vi "Get Next.vi"(0 "Conditional in":refnum<class "Conditional.lvclass">, 1 "Linked List Ref":refnum<data-value>, 5 "Active Unique ID":string, 9 "Active Element Index":i32, 11 "error in (no error)":errorcluster) -> (3 "Linked List Ref out":refnum<data-value>, 4 "Executioner out":refnum<class "Executioner.lvclass">, 6 "Active Unique ID out":string, 8 "Test Executive Ref out":refnum<data-value>, 10 "Active Element Index out":i32, 12 "Found":bool, 13 "Complete":bool, 14 "Stop":bool, 15 "error out":errorcluster)   [LabVIEW 2017, in "Custom Type Test Executive.lvlib" / "Conditional.lvclass"]
uses:
  <vilib>/gpm_packages/@cs/test-executive/Source/Custom Type Test Executive/Conditional/Conditional.lvclass
  C:/Program Files/National Instruments/LabVIEW 2017/vi.lib/gpm_packages/@cs/test-executive/Source/Test Executive/Executioner/Executioner.lvclass
  <vilib>/gpm_packages/@cs/test-executive/Source/Test Executive/Executioner/Executioner.lvclass
  <vilib>/gpm_packages/@cs/linked-list/Source/Linked List/ILinkedList/ILinked List.lvclass
  <vilib>/gpm_packages/@cs/test-executive/Source/Test Executive/ITestExecutive/ITest Executive.lvclass
  <vilib>/gpm_packages/@cs/data-type-serializer/source/String/String.lvclass/String.ctl
  <vilib>/gpm_packages/@cs/data-type-serializer/source/Boolean/Boolean.lvclass/Boolean.ctl
  <vilib>/gpm_packages/@cs/run-time-assertions/Source/Assert/Assert.lvclass
  <vilib>/gpm_packages/@cs/data-type-serializer/source/Assertion/Assertion.lvclass/Assertion.ctl
  3077af34-4ef3-437c-b8d8-6eac68132344.vi
  9cbd8125-b855-42de-ba09-e02fd7405d46.vi
  3190a705-8440-4941-9536-4da4aa80a172.vi
  cabaf482-ba4b-46e4-9c21-873f7cc35bd3.vi
  ea6f5d10-5cf1-43e9-b612-598c02a8f936.vi
  9307d838-b7ae-42de-b3ed-71b38e2b7019.vi
  380485d8-fc70-4f46-821f-d05b1d9706b5.vi
  58626fd2-b79f-420a-b1ac-c7491086ee9c.vi
  da5c0a25-912c-45e8-99a2-8536258bb53a.vi
  193c418e-592a-406e-a7dd-eacb90f55738.vi
  <vilib>/gpm_packages/@cs/data-type-serializer/source/Boolean/Boolean.lvclass
  C:/Program Files/National Instruments/LabVIEW 2017/vi.lib/gpm_packages/@cs/data-type-serializer/source/Data Type/Data Type.lvclass
  <vilib>/gpm_packages/@cs/data-type-serializer/source/Assertion/Assertion.lvclass
  <vilib>/gpm_packages/@cs/data-type-serializer/source/String/String.lvclass
  <vilib>/gpm_packages/@cs/linked-list/Source/Linked List/Linked List Ref/Linked List Ref.lvclass
  <vilib>/gpm_packages/@cs/test-executive/Source/Test Executive/Conditional/Conditional.lvclass
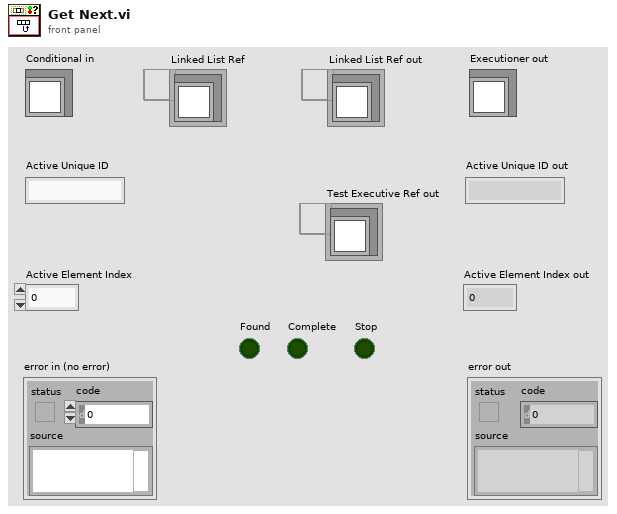
[diagram p1: front panel]
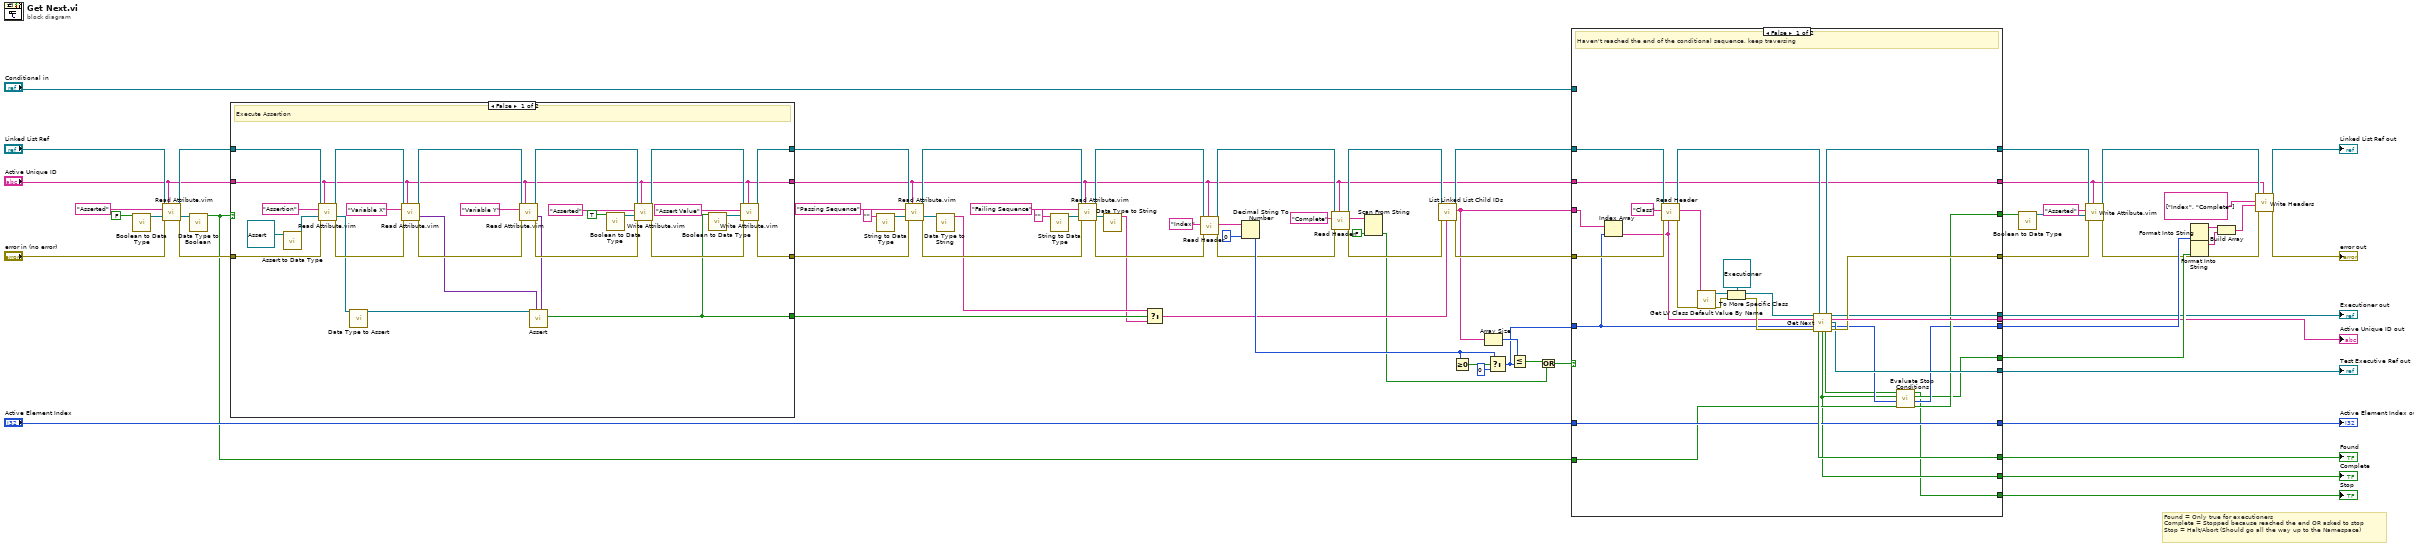
[diagram p0: block diagram]
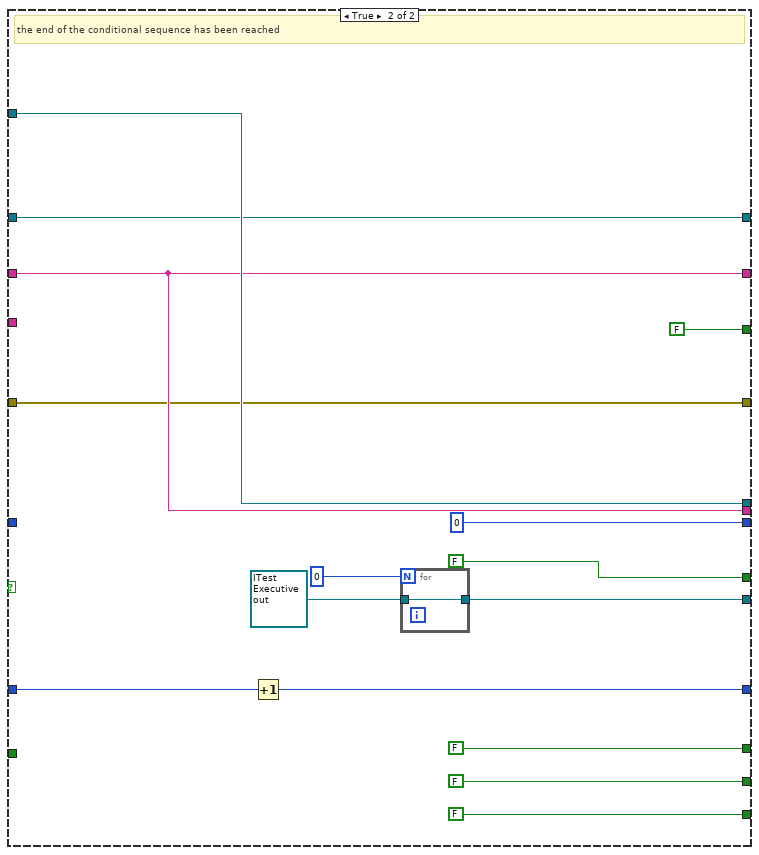
[diagram p2: hidden frame]
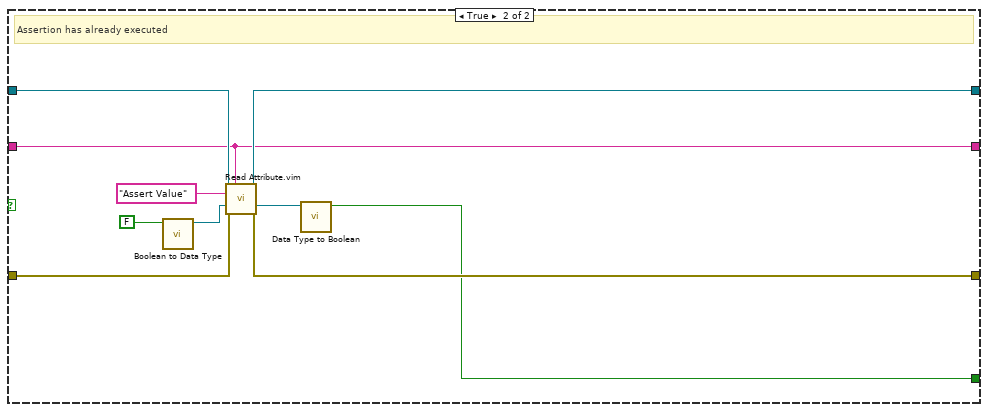
[diagram p3: hidden frame]
diagram:
  # "Found = Only true for executioners\nComplete = Stopped because reached the end OR asked to stop\nStop = Halt/Abort (Should go all the way up to the Namespace)"
  n1 = call <vilib>:"Boolean to Data Type.vi"("Boolean"=FALSE) -> ("Boolean out"=w13:refnum<class "Boolean.lvclass">)  [unwired: 9 in, 1 out]
  n2 = call "Read Attribute.vim"("Linked List Ref"="Linked List Ref", "Linked List ID"="Active Unique ID", "Attribute Name"="Asserted", "Type"=w13, "error in (no error)"="error in (no error)") -> ("Linked List Ref out"=w74:refnum<data-value>, "Attribute"=w12:refnum<class "Boolean.lvclass">, "error out"=w73:errorcluster)  [unwired: 5 in, 3 out]
  n3 = call <vilib>:"Data Type to Boolean.vi"("Data Type"=w12) -> ("Boolean out"=w11:bool)  [unwired: 9 in, 1 out]
  n4 = case shown="False" w11 {
    tunnel: "Active Unique ID" -> [w86 w108]
    tunnel: [w94 w111] -> w71
    tunnel: [w92 w109] -> w72
    tunnel: w74 -> [w98 w112]
    tunnel: w73 -> [w97 w110]
    tunnel: [w77 w106] -> w66
    tunnel: [w86 w108] -> w39
    frame False {
      # "Execute Assertion"
      n5 = call <vilib>:"Assert to Data Type.vi"("Assert"=refnum<class "Assert.lvclass"> refnum ("Run Time Assertions.lvlib:Assert.lvclass")) -> ("Assert out"=w82:refnum<class "Assertion.lvclass">)  [unwired: 9 in, 1 out]
      n6 = call "Read Attribute.vim"("Linked List Ref"=w98, "Linked List ID"=w86, "Attribute Name"="Assertion", "Type"=w82, "error in (no error)"=w97) -> ("Linked List Ref out"=w102:refnum<data-value>, "Attribute"=w81:refnum<class "Assertion.lvclass">, "error out"=w101:errorcluster)  [unwired: 5 in, 3 out]
      n7 = call <vilib>:"Data Type to Assert.vi"("Data Type"=w81) -> ("Assert"=w80:refnum<class "Assert.lvclass">)  [unwired: 9 in, 1 out]
      n8 = call "Read Attribute.vim"("Linked List Ref"=w102, "Linked List ID"=w86, "Attribute Name"="Variable X", "error in (no error)"=w101) -> ("Linked List Ref out"=w89:refnum<data-value>, "Attribute"=w85:variant, "error out"=w90:errorcluster)  [unwired: 6 in, 3 out]
      n9 = call "Read Attribute.vim"("Linked List Ref"=w89, "Linked List ID"=w86, "Attribute Name"="Variable Y", "error in (no error)"=w90) -> ("Linked List Ref out"=w87:refnum<data-value>, "Attribute"=w84:variant, "error out"=w88:errorcluster)  [unwired: 6 in, 3 out]
      n10 = call-dynamic "Assert.vi"("Variable Y"=w84, "Variable X"=w85, "Assert in"=w80) -> ("Assert?"=w77:bool)  [unwired: 8 in]
      n11 = call <vilib>:"Boolean to Data Type.vi"("Boolean"=TRUE) -> ("Boolean out"=w78:refnum<class "Boolean.lvclass">)  [unwired: 9 in, 1 out]
      n12 = call "Write Attribute.vim"("Linked List ID"=w86, "error in (no error)"=w88, "Attribute"=w78, "Attribute Name"="Asserted", "Linked List Ref"=w87) -> ("error out"=w93:errorcluster, "Linked List Ref out"=w95:refnum<data-value>)  [unwired: 3 in, 2 out]
      n13 = call <vilib>:"Boolean to Data Type.vi"("Boolean"=w77) -> ("Boolean out"=w76:refnum<class "Boolean.lvclass">)  [unwired: 9 in, 1 out]
      n14 = call "Write Attribute.vim"("Linked List ID"=w86, "error in (no error)"=w93, "Attribute"=w76, "Attribute Name"="Assert Value", "Linked List Ref"=w95) -> ("error out"=w92:errorcluster, "Linked List Ref out"=w94:refnum<data-value>)  [unwired: 3 in, 2 out]
    }
    frame True {
      # "Assertion has already executed"
      n15 = call <vilib>:"Boolean to Data Type.vi"("Boolean"=FALSE) -> ("Boolean out"=w104:refnum<class "Boolean.lvclass">)  [unwired: 9 in, 1 out]
      n16 = call "Read Attribute.vim"("Linked List Ref"=w112, "Linked List ID"=w108, "Attribute Name"="Assert Value", "Type"=w104, "error in (no error)"=w110) -> ("Linked List Ref out"=w111:refnum<data-value>, "Attribute"=w107:refnum<class "Boolean.lvclass">, "error out"=w109:errorcluster)  [unwired: 5 in, 3 out]
      n17 = call <vilib>:"Data Type to Boolean.vi"("Data Type"=w107) -> ("Boolean out"=w106:bool)  [unwired: 9 in, 1 out]
    }
  }
  n18 = call <vilib>:"String to Data Type.vi"("String"="") -> ("Boolean out"=w9:refnum<class "String.lvclass">)  [unwired: 9 in, 1 out]
  n19 = call "Read Attribute.vim"("Linked List Ref"=w71, "Linked List ID"=w39, "Attribute Name"="Passing Sequence", "Type"=w9, "error in (no error)"=w72) -> ("Linked List Ref out"=w68:refnum<data-value>, "Attribute"=w8:refnum<class "String.lvclass">, "error out"=w67:errorcluster)  [unwired: 5 in, 3 out]
  n20 = call <vilib>:"Data Type to String.vi"("Data Type"=w8) -> ("String out"=w7:string)  [unwired: 9 in, 1 out]
  n21 = call <vilib>:"String to Data Type.vi"("String"="") -> ("Boolean out"=w5:refnum<class "String.lvclass">)  [unwired: 9 in, 1 out]
  n22 = call "Read Attribute.vim"("Linked List Ref"=w68, "Linked List ID"=w39, "Attribute Name"="Failing Sequence", "Type"=w5, "error in (no error)"=w67) -> ("Linked List Ref out"=w65:refnum<data-value>, "Attribute"=w4:refnum<class "String.lvclass">, "error out"=w64:errorcluster)  [unwired: 5 in, 3 out]
  n23 = call <vilib>:"Data Type to String.vi"("Data Type"=w4) -> ("String out"=w3:string)  [unwired: 9 in, 1 out]
  n24 = Select(t=w7, s=w66, f=w3) -> (s? t:f=w54:string)
  n25 = call <vilib>:"Read Header.vi"("Linked List ID"=w39, "error in (no error)"=w64, "Header Name"="Index" ("Attribute Name"), "Linked List Ref"=w65) -> ("error out"=w38:errorcluster, "Header Value"=w51:string, "Linked List Ref out"=w41:refnum<data-value>)  [unwired: 4 in, 1 out]
  n26 = Decimal String To Number(string=w51, default (0L)=0 ("Attribute")) -> (number=w60:i32)  [unwired: 1 in, 1 out]
  n27 = call <vilib>:"Read Header.vi"("Linked List ID"=w39, "error in (no error)"=w38, "Header Name"="Complete" ("Attribute Name"), "Linked List Ref"=w41) -> ("error out"=w37:errorcluster, "Header Value"=w43:string, "Linked List Ref out"=w40:refnum<data-value>)  [unwired: 4 in, 1 out]
  n28 = Scan From String(input string=w43, default 1=FALSE) -> (output 1=w35:bool)  [unwired: 3 in, 3 out]
  n29 = call <vilib>:"List Linked List Child IDs.vi"("Linked List ID"=w54, "error in (no error)"=w37, "Linked List Ref"=w40) -> ("error out"=w58:errorcluster, "Child IDs"=w57:string[], "Linked List Ref out"=w59:refnum<data-value>)  [unwired: 6 in]
  n30 = Greater Or Equal To 0?(x=w60) -> (x >= 0?=w63:bool)
  n31 = Array Size(array=w57) -> (size(s)=w61:i32)
  n32 = Select(t=w60, s=w63, f=0) -> (s? t:f=w56:i32)
  n33 = Less Or Equal?(x=w61, y=w56) -> (x <= y?=w45:bool)
  n34 = Or(x=w45, y=w35) -> (x .or. y?=w36:bool)
  n35 = case shown="False" w36 {
    tunnel: [w134 w146] -> w32
    tunnel: w59 -> [w136 w146]
    tunnel: [w130 w145] -> w30
    tunnel: w58 -> [w138 w145]
    tunnel: w57 -> [w127 _]
    tunnel: w56 -> [w126 _]
    tunnel: [w118 0 ("Active Element Index out")] -> w55
    tunnel: [w122 w155] -> w16
    tunnel: [w133 w151] -> w15
    tunnel: [w132 FALSE ("Found")] -> w20
    tunnel: [w117 FALSE] -> w21
    tunnel: [w114 FALSE] -> w22
    tunnel: "Conditional in" -> [_ w155]
    tunnel: w39 -> [w129 w151]
    tunnel: [w129 w151] -> w29
    tunnel: "Active Element Index" -> [w128 w153]
    tunnel: [w128 w152] -> w19
    tunnel: [w116 FALSE ("Complete")] -> w53
    tunnel: [w124 w147] -> w18
    tunnel: [w120 FALSE] -> w1
    tunnel: w11 -> [w121 _]
    frame False {
      # "Haven't reached the end of the conditional sequence, keep traversing"
      n36 = Index Array(array=w127, index=w126) -> (element=w125:string)
      n37 = call <vilib>:"Read Header.vi"("Linked List ID"=w125, "error in (no error)"=w138, "Header Name"="Class", "Linked List Ref"=w136) -> ("error out"=w131:errorcluster, "Header Value"=w143:string, "Linked List Ref out"=w135:refnum<data-value>)  [unwired: 4 in, 1 out]
      n38 = call <vilib>:"Get LV Class Default Value By Name.vi"("error in (no error)"=w131, "class name"=w143) -> ("error out"=w139:errorcluster, "object"=w142:refnum<class>)  [unwired: 8 in]
      n39 = To More Specific Class(target class=refnum<class "Executioner.lvclass"> refnum ("Test Executive.lvlib:Executioner.lvclass"), reference=w142, error in=w139) -> (specific class reference=w123:refnum<class "Executioner.lvclass">, error out=w140:errorcluster)
      n40 = call-dynamic "Get Next.vi"("Executioner in"=w123, "Linked List Ref"=w135, "Active Unique ID"=w125, "Active Element Index"=w126, "error in (no error)"=w140) -> ("Linked List Ref out"=w134:refnum<data-value>, "Executioner out"=w122:refnum<class "Executioner.lvclass">, "Active Unique ID out"=w133:string, "Test Executive Ref out"=w124:refnum<data-value>, "Active Element Index out"=w119:i32, "Found"=w132:bool, "Complete"=w117:bool, "Stop"=w115:bool, "error out"=w130:errorcluster)  [unwired: 2 in]
      n41 = call <vilib>:"Evaluate Stop Conditions.vi"("Assert"=w121, "Index"=w119, "Complete"=w117, "Stop"=w115) -> ("Asserted"=w120:bool, "Index out"=w118:i32, "Completed"=w116:bool, "Stop out"=w114:bool)  [unwired: 4 in]
    }
    frame True {
      # "the end of the conditional sequence has been reached"
      n42 = Increment(x=w153) -> (x+1=w152:i32)
      n43 = for {
        N: 0 -> [_]
        tunnel: refnum<data-value> refnum ("Test Executive Ref out") -> [w159]
        tunnel: [w159] -> w147
      }
    }
  }
  "Executioner out" <- w16
  "Active Unique ID out" <- w15
  "Active Element Index out" <- w19
  "Found" <- w20
  "Complete" <- w21
  "Stop" <- w22
  "Test Executive Ref out" <- w18
  n44 = call <vilib>:"Boolean to Data Type.vi"("Boolean"=w1) -> ("Boolean out"=w2:refnum<class "Boolean.lvclass">)  [unwired: 9 in, 1 out]
  n45 = call "Write Attribute.vim"("Linked List ID"=w29, "error in (no error)"=w30, "Attribute"=w2, "Attribute Name"="Asserted", "Linked List Ref"=w32) -> ("error out"=w31:errorcluster, "Linked List Ref out"=w33:refnum<data-value>)  [unwired: 3 in, 2 out]
  n46 = Format Into String(w55) -> (resulting string=w48:string)  [unwired: 3 in, 1 out]
  n47 = Format Into String(w53) -> (resulting string=w46:string)  [unwired: 3 in, 1 out]
  n48 = Build Array(w48, w46) -> (w47:string[])
  n49 = call <vilib>:"Write Headers.vi"("Linked List ID"=w29, "error in (no error)"=w31, "Header Values"=w47, "Header Names"=string[] ["Index", "Complete"], "Linked List Ref"=w33) -> ("error out"=→"error out":errorcluster, "Linked List Ref out"=→"Linked List Ref out":refnum<data-value>)  [unwired: 5 in]
